vi "DAQ_E_mIO_DIO.constructor.vi"(0 "name":string, 2 "data in":string, 5 "error in (no error)":errorcluster) -> (14 "i ref out":refnum<vi>, 16 "data out":string, 19 "error out":errorcluster)   [LabVIEW 2014, in "DAQ_E_mIO_DIO.lvlib"]
doc: "constructor of the DAQ_E_mIO_DIO class"
uses:
  DAQ_E_mIO_DIO.lvlib
  CS_Core/CSApplicationBaseClasses/DeviceBase/DeviceBase.myEventNames.ctl
  <vilib>/DAQmx/create/channels.llb/DAQmx Create Channel (DI-Digital Input).vi
  <vilib>/DAQmx/create/channels.llb/DAQmx Create Channel (DO-Digital Output).vi
  CS_Core/CSSystem/CSSystemLib/CSSystemLib.lvlib
  CS_Core/CSApplicationBaseClasses/DigiIOBase/DigiIOBase.lvlib
  CS_Core/CSApplicationBaseClasses/DeviceBase/DeviceBase.lvlib
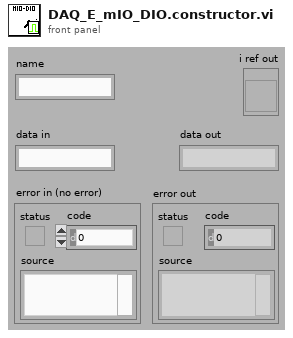
[diagram p1: front panel]
types:
  T1 = enum16{"SetAttribute", "GetAttribute", "CreateAttribute", "DestroyAttribute", "DestroyAllAtributes"}
  T2 = typedef "DeviceBase.lvlib/DeviceBase.myEventNames.ctl" = enum16{"lvmsg://Initialize", "lvmsg://Close", "lvmsg://Configure", "lvmsg://Reset", "lvmsg://IDQuery"}
  T3 = typedef "DAQ_E_mIO_DIO.lvlib/DAQ_E_mIO_DIO.i attribute.ctl" = cluster{"DOutChannel":refnum<k21>, "DInChannel":refnum<k21>, "nOfBitsIn":i32, "nOfBitsOut":i32}
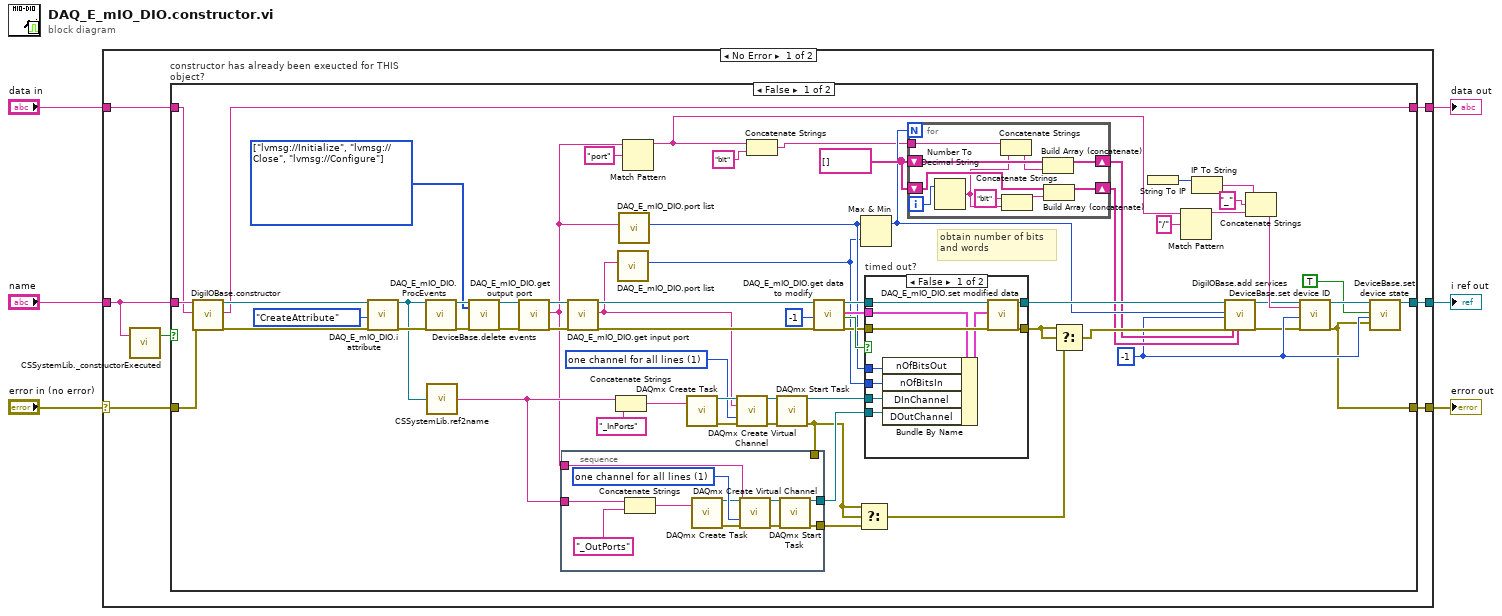
[diagram p0: block diagram]
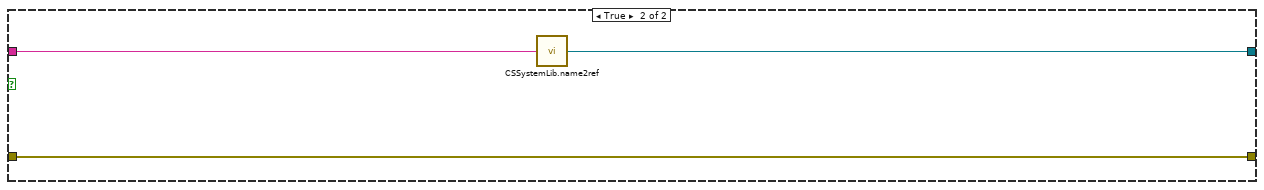
[diagram p3: hidden frame]
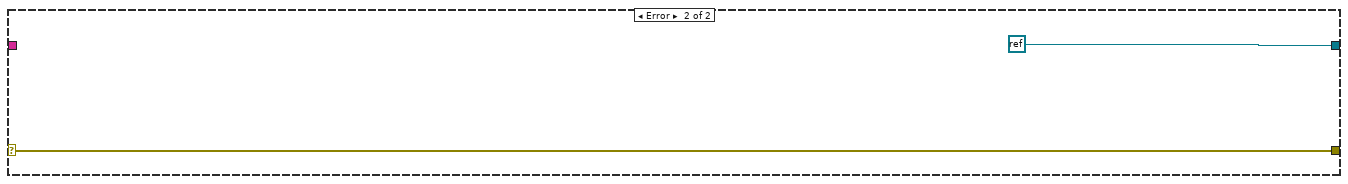
[diagram p4: hidden frame]
diagram:
  n1 = case shown="No Error" "error in (no error)" {
    selector: "error in (no error)" -> [w11 w114]
    tunnel: "name" -> [w9 _]
    tunnel: [w13 refnum<k0> refnum] -> w5
    tunnel: [w12 w114] -> w4
    tunnel: "data in" -> [w8 _]
    tunnel: [w7 _] -> w1
    frame No Error {
      n2 = call "CSSystemLib._constructorExecuted.vi"("name"=w9) -> ("constructor executed?"=w10:bool)  [unwired: 18 in]
      n3 = case "constructor has already been exeucted for THIS object?" shown="False" w10 {
        tunnel: w9 -> [w74 w113]
        tunnel: [w36 w112] -> w13
        tunnel: [w37 w111] -> w12
        tunnel: w11 -> [w49 w111]
        tunnel: w8 -> [w27 _]
        tunnel: [w26 _] -> w7
        frame False {
          w32 = T2[] [enum."lvmsg://Initialize", enum."lvmsg://Close", enum."lvmsg://Configure"] items=["lvmsg://Initialize", "lvmsg://Close", "lvmsg://Configure", "lvmsg://Reset", "lvmsg://IDQuery"] ("events")
          w46 = string[] []
          w39 = -1 ("ms timeout (10000)")
          w70 = 1 items=["one channel for each line", "one channel for all lines"] ("line grouping")
          # "obtain number of bits\nand words"
          n4 = call "DigiIOBase.constructor.vi"("name"=w74, "data in"=w27, "error in (no error)"=w49) -> ("i ref out"=w77:refnum<vi>, "data out"=w26:string, "error out"=w76:errorcluster)  [unwired: 14 in]
          n5 = call "DAQ_E_mIO_DIO.i attribute.vi"("VI Refnum"=w77, "Action"=T1."CreateAttribute", "error in (no error)"=w76) -> ("VI Refnum out"=w56:refnum<vi>, "error out"=w73:errorcluster)  [unwired: 14 in, 1 out]
          n6 = call "DAQ_E_mIO_DIO.ProcEvents.vi"("i ref in"=w56, "error in (no error)"=w73) -> ("i ref out"=w34:refnum<vi>, "error out"=w33:errorcluster)  [unwired: 16 in]
          n7 = call "CSSystemLib.ref2name.vi"("obj refnum"=w56) -> ("name"=w55:string)
          n8 = call "DeviceBase.delete events.vi"("i ref in"=w34, "events"=w32, "error in (no error)"=w33) -> ("i ref out"=w31:refnum<vi>, "error out"=w30:errorcluster)  [unwired: 14 in, 1 out]
          n9 = call "DAQ_E_mIO_DIO.get output port.vi"("i ref in"=w31, "error in (no error)"=w30) -> ("i ref out"=w67:refnum<vi>, "portList"=w22:tag, "error out"=w66:errorcluster)  [unwired: 15 in]
          n10 = call "DAQ_E_mIO_DIO.get input port.vi"("i ref in"=w67, "error in (no error)"=w66) -> ("i ref out"=w65:refnum<vi>, "portList"=w23:tag, "error out"=w64:errorcluster)  [unwired: 15 in]
          n11 = Concatenate Strings(w55, "_InPorts") -> (w54:string)
          n12 = call "DAQ_E_mIO_DIO.port list.vi"("portList"=w23) -> ("nOfBits"=w24:i32)  [unwired: 10 in]
          n13 = call "DAQ_E_mIO_DIO.port list.vi"("portList"=w22) -> ("nOfBits"=w25:i32)  [unwired: 10 in]
          n14 = Match Pattern(string=w22, regular expression="port") -> (before substring=w17:string)  [unwired: 1 in, 3 out]
          n15 = call <vilib>:"DAQmx Create Task.vi"("new task name"=w54) -> ("task out"=w72:refnum<k21>, "error out"=w71:errorcluster)  [unwired: 13 in]
          n16 = call-poly <vilib>:"DAQmx Create Virtual Channel.vi"("task in"=w72, "lines"=w23, "line grouping"=w70, "error in"=w71) -> ("task out"=w68:refnum<k21>, "error out"=w69:errorcluster)  [unwired: 10 in]
          n17 = Concatenate Strings(w17, "bit" ("string")) -> (w15:string)
          n18 = call <vilib>:"DAQmx Start Task.vi"("task/channels in"=w68, "error in"=w69) -> ("task out"=w58:refnum<k21>, "error out"=w35:errorcluster)  [unwired: 12 in]
          n19 = stacked-sequence {
            tunnel: [w93] -> w57
            tunnel: w22 -> [w92]
            tunnel: w55 -> [w91]
            tunnel: [w88] -> w52
            tunnel: w35 -> [_]
            frame #0 {
              w96 = 1 items=["one channel for each line", "one channel for all lines"] ("line grouping")
              n20 = Concatenate Strings(w91, "_OutPorts" ("regular expression (\"\")")) -> (w89:string)
              n21 = call <vilib>:"DAQmx Create Task.vi"("new task name"=w89) -> ("task out"=w94:refnum<k21>, "error out"=w95:errorcluster)  [unwired: 13 in]
              n22 = call-poly <vilib>:"DAQmx Create Virtual Channel.vi"("task in"=w94, "lines"=w92, "line grouping"=w96, "error in"=w95) -> ("task out"=w98:refnum<k21>, "error out"=w97:errorcluster)  [unwired: 10 in]
              n23 = call <vilib>:"DAQmx Start Task.vi"("task/channels in"=w98, "error in"=w97) -> ("task out"=w93:refnum<k21>, "error out"=w88:errorcluster)  [unwired: 12 in]
            }
          }
          n24 = call "DAQ_E_mIO_DIO.get data to modify.vi"("i ref in"=w65, "ms timeout (10000)"=-1, "error in (no error)"=w64) -> ("i ref out"=w61:refnum<vi>, "i attribute"=w59:T3, "timed out"=w62:bool, "error out"=w60:errorcluster)  [unwired: 13 in]
          n25 = Select(t=w35, s=w35, f=w52) -> (s? t:f=w50:errorcluster)
          n26 = Max & Min(x=w25, y=w24) -> (max(x,y)=w45:i32)  [unwired: 1 out]
          n27 = case "timed out?" shown="False" w62 {
            tunnel: [w108 w110] -> w48
            tunnel: w61 -> [w106 w110]
            tunnel: [w107 w109] -> w51
            tunnel: w60 -> [w105 w109]
            tunnel: w59 -> [w104 _]
            tunnel: w58 -> [w102 _]
            tunnel: w57 -> [w101 _]
            tunnel: w25 -> [w100 _]
            tunnel: w24 -> [w99 _]
            frame False {
              n28 = Bundle By Name(cluster=w104, "nOfBitsOut"=w100, "nOfBitsIn"=w99, "DInChannel"=w102, "DOutChannel"=w101) -> (w103:T3)
              n29 = call "DAQ_E_mIO_DIO.set modified data.vi"("i ref in"=w106, "i attribute"=w103, "error in (no error)"=w105) -> ("i ref out"=w108:refnum<vi>, "error out"=w107:errorcluster)  [unwired: 15 in]
            }
            frame True {
            }
          }
          n30 = for {
            N: w45 -> [_]
            shift-right: [w80] -> w44
            shift-left: w46 -> [w87]
            shift-right: [w83] -> w43
            shift-left: w46 -> [w82]
            tunnel: w15 -> [w85]
            i -> [w86]
            n31 = Number To Decimal String(number=w86) -> (decimal integer string=w81:string)  [unwired: 1 in]
            n32 = Concatenate Strings(w85, w81) -> (w84:string)
            n33 = Concatenate Strings("bit" ("string"), w81) -> (w79:string)
            n34 = Build Array (concatenate)(w87, w84) -> (w80:string[])
            n35 = Build Array (concatenate)(w82, w79) -> (w83:string[])
          }
          n36 = Select(t=w51, s=w51, f=w50) -> (s? t:f=w47:errorcluster)
          n37 = String To IP() -> (0:w29:u32)  [unwired: 1 in]
          n38 = Match Pattern(string=w17, regular expression="/") -> (before substring=w18:string)  [unwired: 1 in, 3 out]
          n39 = IP To String(2:w29) -> (0:w28:string)  [unwired: 1 in]
          n40 = call "DigiIOBase.add services.vi"("i ref in"=w48, "nofBits"=w45, "ms timeout (10000)"=w39, "error in (no error)"=w47, "physicalNames"=w44, "logicalNames"=w43) -> ("i ref out"=w20:refnum<vi>, "error out"=w19:errorcluster)  [unwired: 11 in, 1 out]
          n41 = Concatenate Strings(w28, "_" ("string"), w18) -> (w41:string)
          n42 = call "DeviceBase.set device ID.vi"("i ref in"=w20, "deviceID"=w41, "ms timeout (10000)"=w39, "error in (no error)"=w19) -> ("i ref out"=w40:refnum<vi>, "error out"=w37:errorcluster)  [unwired: 13 in, 1 out]
          n43 = call "DeviceBase.set device state.vi"("i ref in"=w40, "implicit"=TRUE, "ms timeout (10000)"=w39, "device error"=w37) -> ("i ref out"=w36:refnum<vi>)  [unwired: 13 in, 2 out]
        }
        frame True {
          n44 = call "CSSystemLib.name2ref.vi"("name"=w113) -> ("obj refnum"=w112:refnum<vi>)
        }
      }
    }
    frame Error {
    }
  }
  "i ref out" <- w5
  "error out" <- w4
  "data out" <- w1
